vi "Сбор Кластеры-02-функции.vi"() -> ()   [LabVIEW 2017]
panel:
  in  "Boolean":bool
  out "Cluster 2":T1
  in  "Cluster":T2
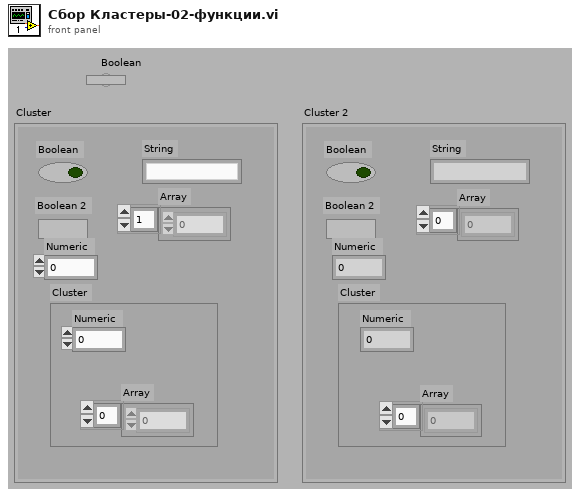
[diagram p1: front panel]
types:
  T1 = cluster{"Array":dbl[], "Cluster":cluster{"Array":u8[], "Numeric":i32}, "Numeric":dbl, "Boolean 2":bool, "String":string, "Boolean":bool}
  T2 = cluster{"Boolean":bool, "Boolean 2":bool, "Numeric":dbl, "String":string, "Array":dbl[], "Cluster":cluster{"Numeric":i32, "Array":u8[]}}
  T3 = cluster{"Array":dbl[], cluster{"Array":u8[], "Numeric":i32}, "Numeric":dbl, "Boolean 2":bool, "String":string, "Boolean":bool}
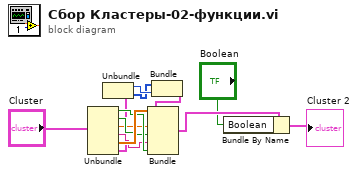
[diagram p0: block diagram]
diagram:
  n1 = Unbundle("Cluster") -> ("Boolean"=w11:bool, "Boolean 2"=w10:bool, "Numeric"=w9:dbl, "String"=w8:string, "Array"=w12:dbl[], "Cluster"=w7:cluster{"Numeric":i32, "Array":u8[]})
  n2 = Unbundle(w7) -> ("Numeric"=w5:i32, "Array"=w4:u8[])
  n3 = Bundle("Array"=w4, "Numeric"=w5) -> (w6:cluster{"Array":u8[], "Numeric":i32})  [unwired: 1 in]
  n4 = Bundle("Array"=w12, w6, "Numeric"=w9, "Boolean 2"=w10, "String"=w8, "Boolean"=w11) -> (w3:T3)  [unwired: 1 in]
  n5 = Bundle By Name(cluster=w3, "Boolean"="Boolean") -> (→"Cluster 2":T3)
